vi "_Main.vi"(10 "Output 2":dbl, 11 "Output":dbl) -> (2 "Output 4":dbl, 3 "Output 3":dbl)   [LabVIEW 2017, in "Claw.lvlib"]
uses:
  Claw.lvlib
  <vilib>/Rock Robotics/SystemInterfaces/DIO/FPGA_DIOPWMChannel.ctl
  <vilib>/Rock Robotics/WPI/MotorControl/WPI_MotorControlOpen Victor.vi
  _SHARE ALL/Global Share All/Global_STOP.vi
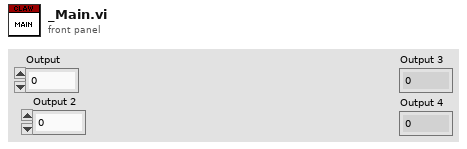
[diagram p1: front panel]
types:
  T1 = typedef "FPGA_DIOPWMChannel.ctl" = enum8{"PWM 0", "PWM 1", "PWM 2", "PWM 3", "PWM 4", "PWM 5", "PWM 6", "PWM 7", "PWM 8", "PWM 9", "PWM MXP 0", "PWM MXP 1", "PWM MXP 2", "PWM MXP 3", "PWM MXP 4", "PWM MXP 5", "PWM MXP 6", "PWM MXP 7", "PWM MXP 8", "PWM MXP 9", "Invalid"}
  T2 = typedef "WPI_MotorControlDeviceRef.ctl" = cluster{"DeviceStatus":errorcluster, "Type":T3, "PWM":cluster{"PWM Channel":T1, "DeadBand":T4}, "CAN":cluster{"Device Number":u8, "SetOutput VI Ref":variant, "GetOutput VI Ref":variant, "Enable VI Ref":variant, "Disable VI Ref":variant, "Data":variant}, "Invert":bool, "DIO PWM":cluster{"PWM \"Enable\" Channel":T1, "DIOChannel":T5, "PWM Rate":dbl}}
  T3 = typedef "WPI_MotorControlType.ctl" = enum16{"PWM", "CAN", "DIO PWM"}
  T4 = typedef "WPI_PWMDeadband.ctl" = cluster{"Name":string, "maxPositivePwm":i32, "minPositivePwm":i32, "centerPwm":i32, "maxNegativePwm":i32, "minNegativePwm":i32, "angularRange":u16}
  T5 = typedef "FPGA_DIOChannel.ctl" = enum8{"DIO 0", "DIO 1", "DIO 2", "DIO 3", "DIO 4", "DIO 5", "DIO 6", "DIO 7", "DIO 8", "DIO 9", "DIO MXP 0", "DIO MXP 1", "DIO MXP 2", "DIO MXP 3", "DIO MXP 4", "DIO MXP 5", "DIO MXP 6", "DIO MXP 7", "DIO MXP 8", "DIO MXP 9", "DIO MXP 10", "DIO MXP 11", "DIO MXP 12", "DIO MXP 13", "DIO MXP 14", "DIO MXP 15", "SPI Port CS1", "SPI Port CS2", "SPI Port CS3", "SPI Port MISO", "SPI Port MOSI", "Invalid"}
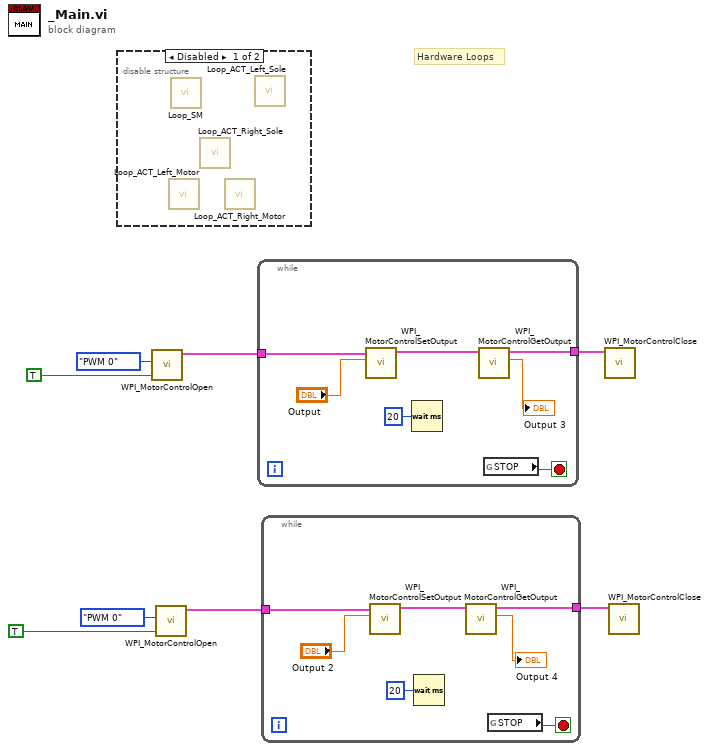
[diagram p0: block diagram]
diagram:
  # "Hardware Loops"
  n1 = disable-structure shown="Disabled" {
    frame Disabled {
      n2 = call "Loop_ACT_Left_Motor.vi"() -> ()  [unwired: 12 in]
      n3 = call "Loop_SM.vi"() -> ()  [unwired: 12 in]
      n4 = call "Loop_ACT_Right_Sole.vi"() -> ()  [unwired: 12 in]
      n5 = call "Loop_ACT_Right_Motor.vi"() -> ()  [unwired: 12 in]
      n6 = call "Loop_ACT_Left_Sole.vi"() -> ()  [unwired: 12 in]
    }
    frame Enabled {
    }
  }
  n7 = call-poly <vilib>:"WPI_MotorControlOpen.vi"("Eliminate Deadband"=TRUE, "PWM Channel"=FPGA_DIOPWMChannel."PWM 0") -> ("MotorControlDeviceRef"=w8:T2)  [unwired: 8 in, 1 out]
  n8 = call-poly <vilib>:"WPI_MotorControlOpen.vi"("Eliminate Deadband"=TRUE, "PWM Channel"=FPGA_DIOPWMChannel."PWM 0") -> ("MotorControlDeviceRef"=w5:T2)  [unwired: 8 in, 1 out]
  n9 = while {
    tunnel: w8 -> [w15]
    tunnel: [w11] -> w7
    stop <- w13 stop-if-true
    n10 = call <vilib>:"WPI_MotorControlSetOutput.vi"("Output"="Output", "MotorControlDevRef"=w15) -> ("MotorControlDevRef"=w12:T2)  [unwired: 7 in, 2 out]
    n11 = Wait (ms)(milliseconds to wait=u32 20) -> ()  [unwired: 1 out]
    n12 = call <vilib>:"WPI_MotorControlGetOutput.vi"("MotorControlDevRef"=w12) -> ("Output"=→"Output 3":dbl, "MotorControlDevRef"=w11:T2)  [unwired: 8 in, 1 out]
    n13 = global read "Global_STOP.vi" "STOP"() -> (w13:bool)
  }
  n14 = while {
    tunnel: w5 -> [w22]
    tunnel: [w18] -> w6
    stop <- w20 stop-if-true
    n15 = call <vilib>:"WPI_MotorControlSetOutput.vi"("Output"="Output 2", "MotorControlDevRef"=w22) -> ("MotorControlDevRef"=w19:T2)  [unwired: 7 in, 2 out]
    n16 = Wait (ms)(milliseconds to wait=u32 20) -> ()  [unwired: 1 out]
    n17 = call <vilib>:"WPI_MotorControlGetOutput.vi"("MotorControlDevRef"=w19) -> ("Output"=→"Output 4":dbl, "MotorControlDevRef"=w18:T2)  [unwired: 8 in, 1 out]
    n18 = global read "Global_STOP.vi" "STOP"() -> (w20:bool)
  }
  n19 = call <vilib>:"WPI_MotorControlClose.vi"("MotorControlDevRef"=w7) -> ()  [unwired: 10 in, 1 out]
  n20 = call <vilib>:"WPI_MotorControlClose.vi"("MotorControlDevRef"=w6) -> ()  [unwired: 10 in, 1 out]
